vi "Set Logging Level.vi"(8 "error in (no error)":errorcluster, 9 "Logging Level":T1) -> (0 "error out":errorcluster)   [LabVIEW 2019, in "Logger.lvlib" / "Logger.lvclass"]
uses:
  Logger.lvclass
  Type Defs/Logging Level.ctl
  Global Variables/Logging Configuration.vi
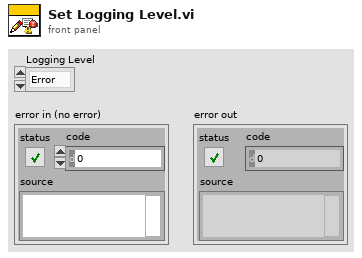
[diagram p1: front panel]
types:
  T1 = typedef "Logger.lvlib/Logger.lvclass/Logging Level.ctl" = enum16{"Error", "Warning", "Info", "Trace"}
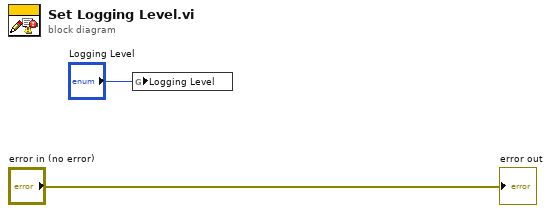
[diagram p0: block diagram]
diagram:
  n1 = global write "Logging Configuration.vi" "Logging Level"("Logging Level") -> ()
  "error out" <- "error in (no error)"
